vi "PeriodicDBsave.vi"(6 "Check pace (sec)":dbl=5.0, 8 "error in (no error)":errorcluster, 11 "FAMM in":refnum<class "FAMM.lvclass">) -> (0 "error out":errorcluster, 3 "FAMM out":refnum<class "FAMM.lvclass">)   [LabVIEW 2014, in "FAMM.lvclass"]
doc: "Periodic check if data has to be saved to the database,\nthe pace input defines the inteval at which the data memory is saved."
uses:
  FAMM.lvclass
  DBAL/DBAL.lvclass
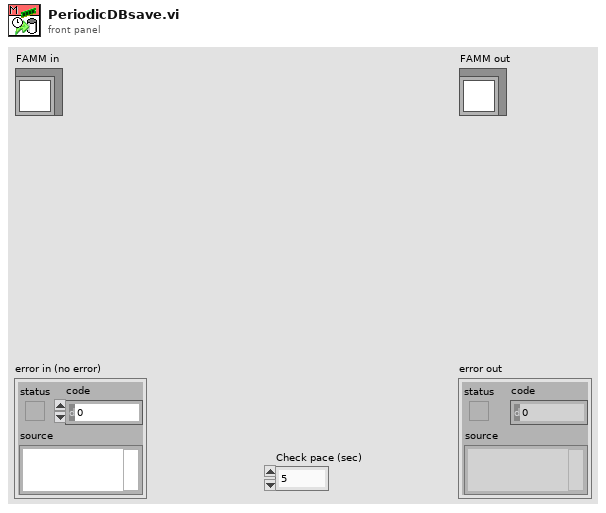
[diagram p1: front panel]
types:
  T1 = cluster{"TableName":string, "Data2save":cluster{"TAGs":string[], "time":dbl[], "TagsData":cluster{"data":dbl[], "max":dbl[], "min":dbl[], "status":u32[]}[]}}[]
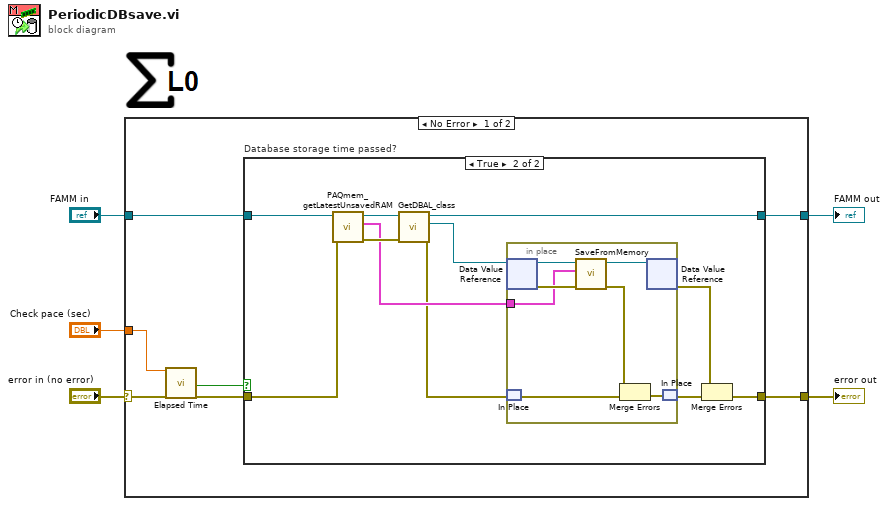
[diagram p0: block diagram]
diagram:
  n1 = case shown="No Error" "error in (no error)" {
    selector: "error in (no error)" -> [w9 w34]
    tunnel: [w7 w34] -> w4
    tunnel: [w10 w33] -> w2
    tunnel: "FAMM in" -> [w11 w33]
    tunnel: "Check pace (sec)" -> [w6 _]
    frame No Error {
      n2 = call "Elapsed Time"("Time Target (s)"=w6, "error in (no error)"=w9) -> ("Time has Elapsed"=w12:bool, "error out"=w8:errorcluster)  [unwired: 10 in, 6 out]
      n3 = case "Database storage time passed?" shown="True" w12 {
        tunnel: w11 -> [w14 w25]
        tunnel: [w14 w22] -> w10
        tunnel: w8 -> [w13 w24]
        tunnel: [w13 w15] -> w7
        frame False {
        }
        frame True {
          n4 = call "PAQmem_getLatestUnsavedRAM.vi"("error in (no error)"=w24, "FAMM in"=w25) -> ("error out"=w21:errorcluster, "Data_2_Save"=w19:T1, "FAMM out"=w23:refnum<class "FAMM.lvclass">)  [unwired: 7 in]
          n5 = call "GetDBAL_class.vi"("error in (no error)"=w21, "FAMM in"=w23) -> ("error out"=w18:errorcluster, "DBAL_class"=w20:refnum<data-value>, "FAMM out"=w22:refnum<class "FAMM.lvclass">)  [unwired: 7 in]
          n6 = in-place {
            in-place-border: w19 -> [w29]
            n7 = in-place-dvr #1(w20) -> (w32:refnum<class "DBAL.lvclass">, w30:errorcluster)
            n8 = in-place-match #2(w18) -> (w28:errorcluster)
            n9 = call-dynamic "SaveFromMemory.vi"("error in (no error)"=w30, "Data_2_Save"=w29, "DBAL in"=w32) -> ("error out"=w27:errorcluster, "DBAL out"=w31:refnum<class "DBAL.lvclass">)  [unwired: 7 in]
            n10 = Merge Errors(w27, w28) -> (w26:errorcluster)
            n11 = in-place-dvr #1(w31) -> (w17:errorcluster)  [unwired: 1 out]
            n12 = in-place-match #2(w26) -> (w16:errorcluster)
          }
          n13 = Merge Errors(w17, w16) -> (w15:errorcluster)
        }
      }
    }
    frame Error {
    }
  }
  "error out" <- w4
  "FAMM out" <- w2
